vi "Pre-Build Action.vi"(6 "Top Level/Always Included VIs":path[](array[path]), 7 "Main Destination Path":path, 9 "Target Name":string, 10 "Build Specification Name":string, 11 "Project Path":path) -> (0 "error out":errorcluster)   [LabVIEW 2023]
uses:
  <vilib>/AppBuilder/AB_API_Simple/Build Specification Version.ctl
  <vilib>/AppBuilder/AB_API_Simple/Set Build Specification Version (path).vi
  <vilib>/AppBuilder/AB_API_Simple/NI_App_Builder_API.lvlib
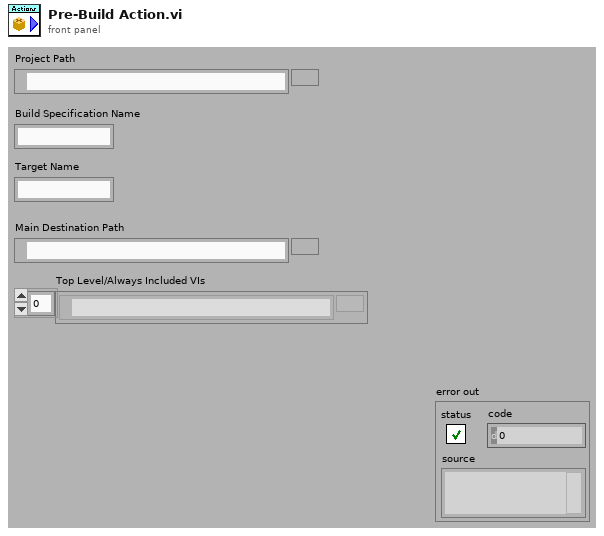
[diagram p1: front panel]
types:
  T1 = typedef "NI_App_Builder_API.lvlib/Build Specification Version.ctl" = cluster{"Major":u16, "Minor":u16, "Fix":u16, "Build":u16}
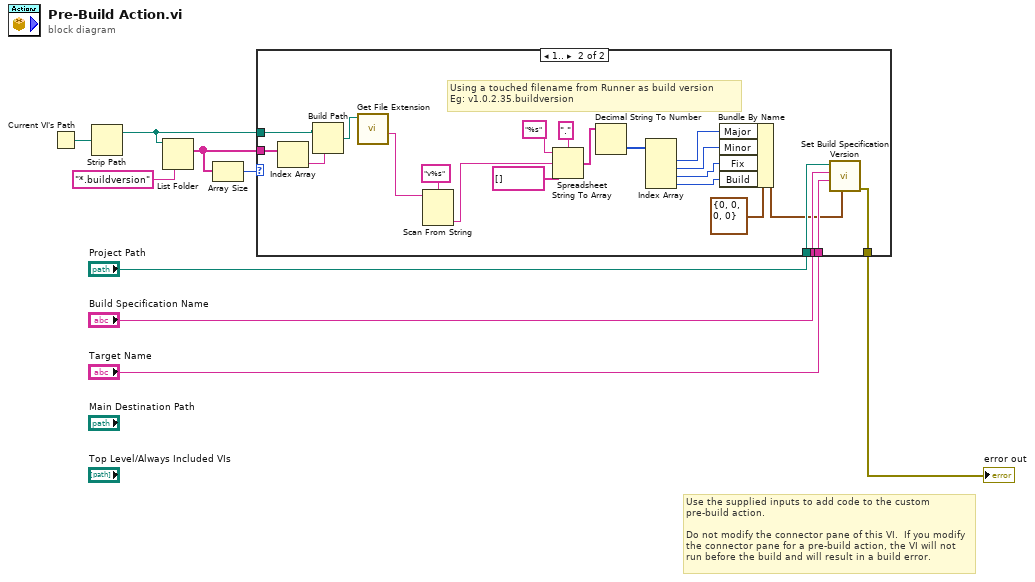
[diagram p0: block diagram]
diagram:
  # "Use the supplied inputs to add code to the custom pre-build action.\n\nDo not modify the connector pane of this VI.  If you modify the connector pane for a pre-build action, the VI will not run before the build and will result in a build error."
  n1 = Current VI's Path() -> (path=w5:path)
  n2 = Strip Path(path=w5) -> (stripped path=w3:path)  [unwired: 1 out]
  n3 = List Folder(path=w3, pattern="*.buildversion") -> (filenames=w2:string[])  [unwired: 2 in, 3 out]
  n4 = Array Size(array=w2) -> (size(s)=w1:i32)
  n5 = case shown="1.." w1 {
    tunnel: [_ w31] -> w9
    tunnel: "Build Specification Name" -> [_ w30]
    tunnel: "Project Path" -> [_ w29]
    tunnel: "Target Name" -> [_ w28]
    tunnel: w2 -> [_ w27]
    tunnel: w3 -> [_ w12]
    frame 0, Default {
    }
    frame 1.. {
      # "Using a touched filename from Runner as build version\nEg: v1.0.2.35.buildversion"
      n6 = Index Array(array=w27) -> (element=w11:string)  [unwired: 1 in]
      n7 = Build Path(base path=w12, name or relative path=w11) -> (appended path=w13:path)
      n8 = call <vilib>:"Get File Extension.vi"("file"=w13) -> ("filename without extension"=w10:string)  [unwired: 6 in, 4 out]
      n9 = Scan From String(format string="v%s", input string=w10) -> (output 1=w14:string)  [unwired: 3 in, 3 out]
      n10 = Spreadsheet String To Array(delimiter (Tab)=".", format string="%s", spreadsheet string=w14, array type (2D Dbl)=string[] []) -> (array=w21:string[])
      n11 = Decimal String To Number(string=w21) -> (number=w20:i32[])  [unwired: 2 in, 1 out]
      n12 = Index Array(array=w20) -> (element #1=w19:i32, element #2=w18:i32, element #3=w17:i32, element #4=w16:i32)  [unwired: 4 in]
      n13 = Bundle By Name(cluster=T1 {"Major"=0, "Minor"=0, "Fix"=0, "Build"=0} ("Build Specification Version"), "Major"=w19, "Minor"=w18, "Fix"=w17, "Build"=w16) -> (w22:T1)
      n14 = call-poly <vilib>:"Set Build Specification Version.vi"("Build Specification Version"=w22, "Name of target (My Computer)"=w28, "Name of build specification"=w30, "Path to project"=w29) -> ("error out"=w31:errorcluster)  [unwired: 7 in]
    }
  }
  "error out" <- w9
